vi "receiveEvent.vi"(8 "error in (no error)":errorcluster, 10 "data":refnum<class>, 11 "ScriptEvent in":refnum<class "ScriptEvent.lvclass">) -> (0 "error out":errorcluster, 2 "Event Type":enum16{"Open", "Save", "Close", "Unregistered"}(ring), 3 "ScriptEvent out":refnum<class "ScriptEvent.lvclass">)   [LabVIEW 2011, in "Events.lvlib" / "ScriptEvent.lvclass"]
uses:
  ScriptEvent.lvclass
  ScriptEvent.lvclass/ScriptEvent.ctl
  Event.lvclass
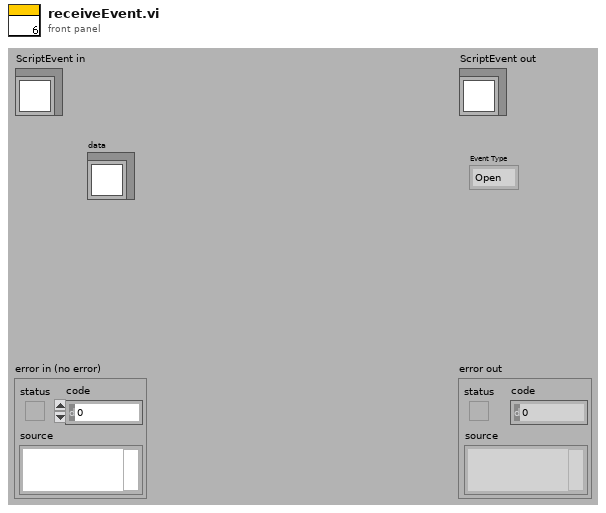
[diagram p1: front panel]
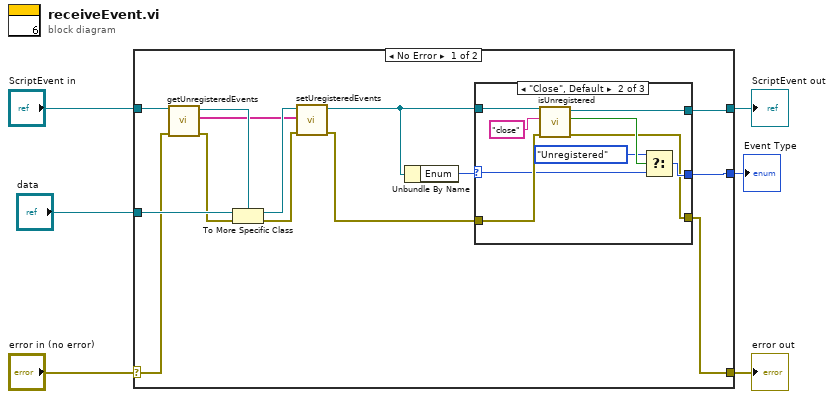
[diagram p0: block diagram]
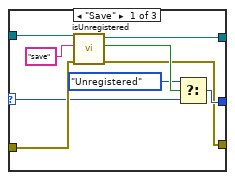
[diagram p2: hidden frame]
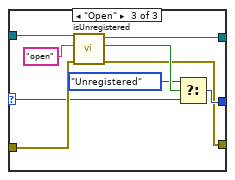
[diagram p3: hidden frame]
diagram:
  n1 = case shown="No Error" "error in (no error)" {
    selector: "error in (no error)" -> [w7 w49]
    tunnel: [w17 w49] -> w5
    tunnel: [w19 w48] -> w3
    tunnel: "ScriptEvent in" -> [w15 w48]
    tunnel: "data" -> [w20 _]
    tunnel: [w18 _] -> w1
    frame No Error {
      n2 = call "getUnregisteredEvents.vi"("error in (no error)"=w7, "Event.lvclass in"=w15) -> ("error out"=w8:errorcluster, "unregisteredEvents"=w12:string[], "Event.lvclass out"=w14:refnum<class "ScriptEvent.lvclass">)  [unwired: 7 in]
      n3 = To More Specific Class(target class=w14, reference=w20, error in=w8) -> (specific class reference=w13:refnum<class "ScriptEvent.lvclass">, error out=w10:errorcluster)
      n4 = call "setUregisteredEvents.vi"("error in (no error)"=w10, "unregisteredEvents"=w12, "Event.lvclass in"=w13) -> ("error out"=w9:errorcluster, "Event.lvclass out"=w11:refnum<class "ScriptEvent.lvclass">)  [unwired: 7 in]
      n5 = Unbundle By Name(w11) -> ("Enum"=w16:enum16{"Open", "Save", "Close", "Unregistered"})
      n6 = case shown="\"Close\", Default" w16 {
        selector: w16 -> [w23 w32 w41]
        tunnel: w11 -> [w29 w38 w47]
        tunnel: [w28 w37 w46] -> w19
        tunnel: w9 -> [w26 w35 w44]
        tunnel: [w22 w31 w40] -> w18
        tunnel: [w21 w30 w39] -> w17
        frame "Save" {
          n7 = call "isUnregistered.vi"("error in (no error)"=w26, "name"="save", "Event in"=w29) -> ("error out"=w21:errorcluster, "unregistered"=w25:bool, "Event out"=w28:refnum<class "ScriptEvent.lvclass">)  [unwired: 6 in]
          n8 = Select(t=enum16{"Open", "Save", "Close", "Unregistered"}."Unregistered" ("Enum"), s=w25, f=w23) -> (s? t:f=w22:enum16{"Open", "Save", "Close", "Unregistered"})
        }
        frame "Close", Default {
          n9 = call "isUnregistered.vi"("error in (no error)"=w35, "name"="close", "Event in"=w38) -> ("error out"=w30:errorcluster, "unregistered"=w34:bool, "Event out"=w37:refnum<class "ScriptEvent.lvclass">)  [unwired: 6 in]
          n10 = Select(t=enum16{"Open", "Save", "Close", "Unregistered"}."Unregistered" ("Enum"), s=w34, f=w32) -> (s? t:f=w31:enum16{"Open", "Save", "Close", "Unregistered"})
        }
        frame "Open" {
          n11 = call "isUnregistered.vi"("error in (no error)"=w44, "name"="open", "Event in"=w47) -> ("error out"=w39:errorcluster, "unregistered"=w43:bool, "Event out"=w46:refnum<class "ScriptEvent.lvclass">)  [unwired: 6 in]
          n12 = Select(t=enum16{"Open", "Save", "Close", "Unregistered"}."Unregistered" ("Enum"), s=w43, f=w41) -> (s? t:f=w40:enum16{"Open", "Save", "Close", "Unregistered"})
        }
      }
    }
    frame Error {
    }
  }
  "error out" <- w5
  "ScriptEvent out" <- w3
  "Event Type" <- w1
